vi "Do.vi"(8 "error in (no error)":errorcluster, 10 "Actor in":refnum<class "Actor.lvclass">, 11 "Message":refnum<class "Request Iteration Notification Msg.lvclass">) -> (0 "error out":errorcluster, 2 "Actor out":refnum<class "Actor.lvclass">)   [LabVIEW 2023, in "Iterator Actor.lvlib" / "Request Iteration Notification Msg.lvclass"]
doc: "(<B>Filename</B>: Actor Framework.lvlib:Reply Msg.lvclass:Do Core.vi)\n\nDefines what an actor does when it receives <B>Reply Message</B>. This method also defines the <B>Reply</B> that is returned to the actor that sent <B>Reply Message</B>.\n\nBy default, this method does nothing, and <B>Reply</B> is the ancestor Message class. A child class must override this method to define behavior and specify a child of the Message class to return in the <B>Reply</B> output."
uses:
  Request Iteration Notification Msg.lvclass
  <vilib>/ActorFramework/Actor/Actor.lvclass
  Request Iteration Notification Msg.lvclass/Request Iteration Notification Msg.ctl
  Notify Iteration Msg/Notify Iteration Msg.lvclass
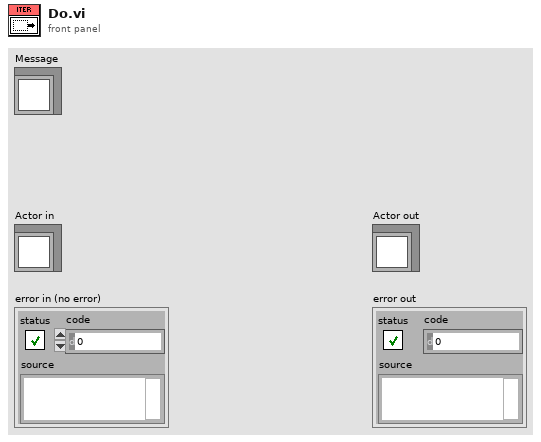
[diagram p1: front panel]
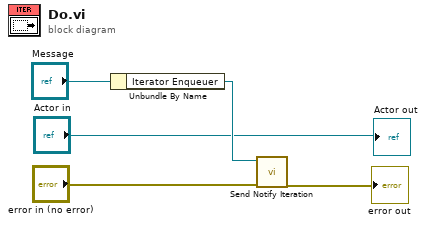
[diagram p0: block diagram]
diagram:
  n1 = Unbundle By Name("Message") -> ("Iterator Enqueuer"=w4:refnum<class "Message Enqueuer.lvclass">)
  n2 = call "Send Notify Iteration.vi"("error in (no error)"="error in (no error)", "Message Enqueuer in"=w4) -> ("error out"=→"error out":errorcluster)  [unwired: 8 in, 1 out]
  "Actor out" <- "Actor in"
